vi "Chocolate Station Keep.vi"(8 "reinitialize":bool) -> (0 "right P.V.":dbl, 1 "right setpoint":dbl, 2 "left P.V.":dbl, 3 "left setpoint":dbl)   [LabVIEW 2011]
uses:
  <vilib>/addons/control/pid/pid.llb/PID (DBL).vi
  <vilib>/addons/control/pid/NI_PID_pid.lvlib
panel:
  out "right":dbl
  out "left":dbl
  in  "Right PID gains":T1={"proportional gain (Kc)"=0.15, "integral time (Ti, min)"=10.0, "derivative time (Td, min)"=0.0} {"derivative time (Td, min)" format="%.3f"; "integral time (Ti, min)" format="%.3f"; "proportional gain (Kc)" format="%.3f"}
  in  "Left PID gains":T1={"proportional gain (Kc)"=0.15, "integral time (Ti, min)"=10.0, "derivative time (Td, min)"=0.0} {"derivative time (Td, min)" format="%.3f"; "integral time (Ti, min)" format="%.3f"; "proportional gain (Kc)" format="%.3f"}
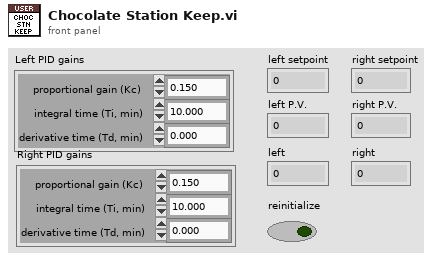
[diagram p1: front panel]
types:
  T1 = cluster{"proportional gain (Kc)":dbl, "integral time (Ti, min)":dbl, "derivative time (Td, min)":dbl}
  T2 = typedef "WPI_RobotDriveDevRef.ctl" = cluster{"DevStatus":errorcluster, "Motors[]":T3[], "Square Inputs":bool, "Max Output":dbl, "Isochronous":bool}
  T3 = typedef "WPI_MotorControlDeviceRef.ctl" = cluster{"DeviceStatus":errorcluster, "Type":enum16{"PWM", "CAN"}, "PWM":cluster{"Digital Module":T4, "PWM Channel":T5, "DeadBand":T6}, "CAN":cluster{"Device Number":u8, "Control Mode":T7, "Semaphore":T8, "Max Vout":dbl}, "Invert":bool, "TransformRef":T9, "InvTransformRef":T9}
  T4 = typedef "FPGA_TypedefDigitalModule.ctl" = enum16{"Digital Module 1", "Digital Module 2"}
  T5 = typedef "FPGA_DIOPWMChannel.ctl" = enum8{"PWM 1", "PWM 2", "PWM 3", "PWM 4", "PWM 5", "PWM 6", "PWM 7", "PWM 8", "PWM 9", "PWM 10", "Invalid"}
  T6 = typedef "WPI_PWMDeadband.ctl" = cluster{"Name":string, "maxPositivePwm":i32, "minPositivePwm":i32, "centerPwm":i32, "maxNegativePwm":i32, "minNegativePwm":i32, "angularRange":u16}
  T7 = typedef "WPI_CANJaguar_ControlMode.ctl" = enum8{"Percent VBus", "Current", "Speed", "Position", "Voltage"}
  T8 = typedef "Semaphore RefNum" = refnum<k1>
  T9 = typedef "WPI_PWMTransform_ConPane.ctl" = refnum<vi>
  T10 = typedef "WPI_JoystickDevRef.ctl" = cluster{"Device":T11}
  T11 = typedef "WPI_JoystickDeviceEnum.ctl" = enum16{"USB 1", "USB 2", "USB 3", "USB 4", "Kinect 1", "Kinect 2"}
  T12 = typedef "WPI_EncoderDevRef.ctl" = cluster{"DevStatus":errorcluster, "EncoderIndex":T13, "CounterIndex":T14, "DistancePerCount":dbl, "Decoding Type":T15}
  T13 = typedef "FPGA_EncoderIdx.ctl" = enum8{"Enc 0", "Enc 1", "Enc 2", "Enc 3", "Invalid"}
  T14 = typedef "FPGA_CounterCtrSystemIndex.ctl" = enum8{"Ctr 0", "Ctr 1", "Ctr 2", "Ctr 3", "Ctr 4", "Ctr 5", "Ctr 6", "Ctr 7", "Invalid"}
  T15 = typedef "WPI_EncoderType.ctl" = enum16{"1x", "2x", "4x"}
  T16 = cluster{"axis 1 (x)":dbl, "axis 2 (y)":dbl, "axis 3 (throttle)":dbl, "axis 4":dbl, "axis 5":dbl, "axis 6":dbl}
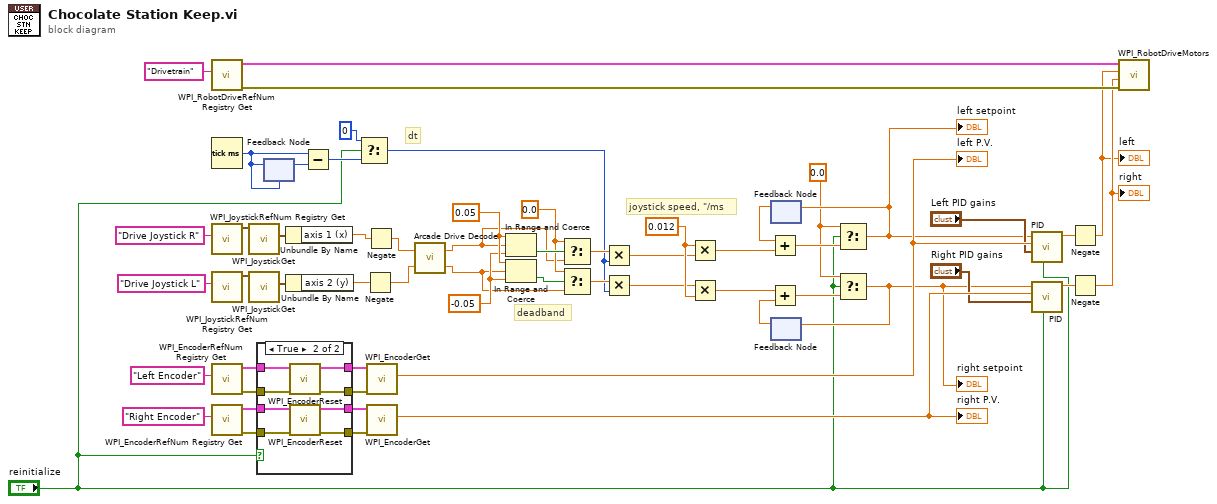
[diagram p0: block diagram]
diagram:
  w13 = 0.012 ("x")
  w23 = 0.0 ("t")
  w25 = -0.05 ("lower limit")
  w26 = 0.05 ("upper limit")
  w32 = 0.0 ("t")
  # "dt"
  # "joystick speed, \"/ms"
  # "deadband"
  n1 = call <vilib>:"WPI_RobotDriveRefNum Registry Get.vi"("refnum name"="Drivetrain") -> ("error out"=w27:errorcluster, "RobotDriveDevRef"=w28:T2)  [unwired: 9 in]
  n2 = Tick Count (ms)() -> (millisecond timer value=w31:u32)
  n3 = call <vilib>:"WPI_JoystickRefNum Registry Get.vi"("refnum name"="Drive Joystick R") -> ("JoystickDevRef"=w56:T10)  [unwired: 9 in, 1 out]
  n4 = call <vilib>:"WPI_JoystickRefNum Registry Get.vi"("refnum name"="Drive Joystick L") -> ("JoystickDevRef"=w55:T10)  [unwired: 9 in, 1 out]
  n5 = call <vilib>:"WPI_EncoderRefNum Registry Get.vi"("refnum name"="Left Encoder") -> ("error out"=w46:errorcluster, "EncoderDevRef"=w48:T12)  [unwired: 9 in]
  n6 = call <vilib>:"WPI_EncoderRefNum Registry Get.vi"("refnum name"="Right Encoder") -> ("error out"=w45:errorcluster, "EncoderDevRef"=w47:T12)  [unwired: 9 in]
  n7 = call <vilib>:"WPI_JoystickGet.vi"("JoystickDevRef"=w56) -> ("Axes"=w54:T16)  [unwired: 4 in, 2 out]
  n8 = call <vilib>:"WPI_JoystickGet.vi"("JoystickDevRef"=w55) -> ("Axes"=w53:T16)  [unwired: 4 in, 2 out]
  n9 = case shown="True" "reinitialize" {
    tunnel: w48 -> [w62 w67]
    tunnel: w47 -> [w60 w63]
    tunnel: w46 -> [w61 w70]
    tunnel: w45 -> [w59 w66]
    tunnel: [w62 w68] -> w44
    tunnel: [w61 w69] -> w43
    tunnel: [w60 w64] -> w42
    tunnel: [w59 w65] -> w41
    frame False {
    }
    frame True {
      n10 = call <vilib>:"WPI_EncoderReset.vi"("error in (no error)"=w70, "EncoderDevRef"=w67) -> ("error out"=w69:errorcluster, "EncoderDevRef"=w68:T12)  [unwired: 8 in]
      n11 = call <vilib>:"WPI_EncoderReset.vi"("error in (no error)"=w66, "EncoderDevRef"=w63) -> ("error out"=w65:errorcluster, "EncoderDevRef"=w64:T12)  [unwired: 8 in]
    }
  }
  n12 = feedback-in #1(w31) -> ()
  n13 = feedback #1(w31) -> (w30:u32)
  n14 = Unbundle By Name(w54) -> ("axis 1 (x)"=w6:dbl)
  n15 = Unbundle By Name(w53) -> ("axis 2 (y)"=w19:dbl)
  n16 = Subtract(x=w31, y=w30) -> (x-y=w4:u32)
  n17 = Select(t=u32 0, s="reinitialize", f=w4) -> (s? t:f=w2:u32)
  n18 = Negate(x=w19) -> (-x=w18:dbl)
  n19 = Negate(x=w6) -> (-x=w5:dbl)
  n20 = call <vilib>:"WPI_EncoderGet.vi"("error in (no error)"=w43, "EncoderDevRef"=w44) -> ("Distance"=w40:dbl)  [unwired: 4 in, 5 out]
  "left P.V." <- w40
  n21 = call <vilib>:"WPI_EncoderGet.vi"("error in (no error)"=w41, "EncoderDevRef"=w42) -> ("Distance"=w39:dbl)  [unwired: 4 in, 5 out]
  "right P.V." <- w39
  n22 = call "Arcade Drive Decode.vi"("Y axis value"=w18, "X axis value"=w5) -> ("Right speed"=w20:dbl, "Left speed"=w21:dbl)
  n23 = In Range and Coerce(upper limit=w26, x=w21, lower limit=w25) -> (In Range?=w24:bool)  [unwired: 1 out]
  n24 = In Range and Coerce(upper limit=w26, x=w20, lower limit=w25) -> (In Range?=w22:bool)  [unwired: 1 out]
  n25 = Select(t=w23, s=w24, f=w21) -> (s? t:f=w12:dbl)
  n26 = Select(t=w23, s=w22, f=w20) -> (s? t:f=w11:dbl)
  n27 = Multiply(x=w12, y=w2) -> (x*y=w10:dbl)
  n28 = Multiply(x=w11, y=w2) -> (x*y=w7:dbl)
  n29 = Multiply(x=w13, y=w10) -> (x*y=w9:dbl)
  n30 = Multiply(x=w7, y=w13) -> (x*y=w8:dbl)
  n31 = feedback #2() -> (w52:dbl)  [unwired: 1 in]
  n32 = Add(x=w52, y=w9) -> (x+y=w35:dbl)
  n33 = feedback #3() -> (w51:dbl)  [unwired: 1 in]
  n34 = Add(x=w8, y=w51) -> (x+y=w33:dbl)
  n35 = Select(t=w32, s="reinitialize", f=w35) -> (s? t:f=w36:dbl)
  "left setpoint" <- w36
  n36 = feedback-in #2(w36) -> ()
  n37 = Select(t=w32, s="reinitialize", f=w33) -> (s? t:f=w34:dbl)
  "right setpoint" <- w34
  n38 = feedback-in #3(w34) -> ()
  n39 = call-poly <vilib>:"PID.vi"("reinitialize? (F)"="reinitialize", "PID gains"="Left PID gains", "process variable"=w40, "setpoint"=w36) -> ("output"=w15:dbl)  [unwired: 6 in, 1 out]
  n40 = call-poly <vilib>:"PID.vi"("reinitialize? (F)"="reinitialize", "PID gains"="Right PID gains", "process variable"=w39, "setpoint"=w34) -> ("output"=w17:dbl)  [unwired: 6 in, 1 out]
  n41 = Negate(x=w15) -> (-x=w14:dbl)
  "left" <- w14
  n42 = Negate(x=w17) -> (-x=w16:dbl)
  "right" <- w16
  n43 = call <vilib>:"WPI_RobotDriveMotors.vi"("error in (no error)"=w27, "RightSpeed"=w16, "LeftSpeed"=w14, "RobotDriveDevRef"=w28) -> ()  [unwired: 6 in, 2 out]
